vi "Subvi(concept).vi"() -> ()   [LabVIEW 2019]
panel:
  in  "stop":bool
  out "Temp in K":dbl
  out "Temp in F":dbl
  in  "Temp in C":dbl
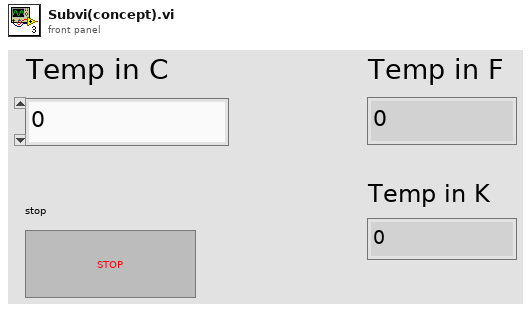
[diagram p1: front panel]
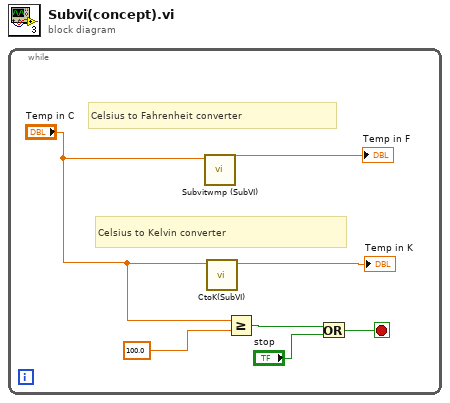
[diagram p0: block diagram]
diagram:
  n1 = while {
    stop <- w1 stop-if-true
    # "Celsius to Kelvin converter"
    # "Celsius to Fahrenheit converter"
    n2 = call "Subvitwmp (SubVI).vi"("Temp in C"="Temp in C") -> ("Temp in F"=→"Temp in F":dbl)  [unwired: 10 in]
    n3 = call "CtoK(SubVI).vi"("Temp in C"="Temp in C") -> ("Numeric"=→"Temp in K":dbl)  [unwired: 10 in]
    n4 = Greater Or Equal?(x="Temp in C", y=100.0) -> (x >= y?=w4:bool)
    n5 = Or(x=w4, y="stop") -> (x .or. y?=w1:bool)
  }
